vi "RamdomCOlumsFileio.vi"   [LabVIEW 2015]
types:
  T1 = enum16{"open", "replace", "create", "open or create", "replace or create", "replace or create with confirmation"}
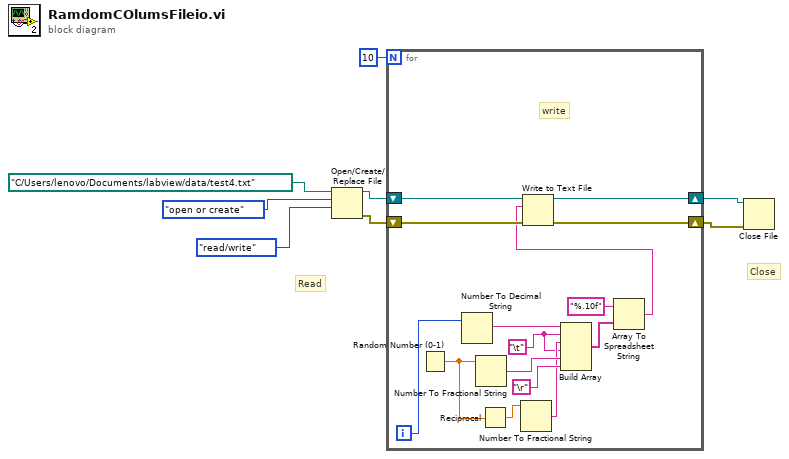
[diagram p0: block diagram]
diagram:
  # "Read"
  # "Close"
  n1 = Open/Create/Replace File(file path (use dialog)=path "C:/Users/lenovo/Documents/labview/data/test4.txt", operation (0:open)=T1."open or create", access (0:read/write)=enum16{"read/write", "read-only", "write-only"}."read/write") -> (refnum out=w4:refnum<file>, error out=w3:errorcluster)  [unwired: 3 in, 1 out]
  n2 = for {
    N: 10 -> [_]
    shift-right: [w20] -> w1
    shift-left: w4 -> [w23]
    shift-right: [w21] -> w2
    shift-left: w3 -> [w22]
    i -> [w18]
    w9 = "\t"
    # "write"
    n3 = Random Number (0-1)() -> (number: 0 to 1=w11:dbl)
    n4 = Number To Decimal String(number=w18) -> (decimal integer string=w19:string)  [unwired: 1 in]
    n5 = Number To Fractional String(number=w11) -> (F-format string=w13:string)  [unwired: 3 in]
    n6 = Reciprocal(x=w11) -> (1/x=w12:dbl)
    n7 = Number To Fractional String(number=w12) -> (F-format string=w10:string)  [unwired: 3 in]
    n8 = Build Array(w19, w9, w10, w9, w13, "\r") -> (w16:string[])
    n9 = Array To Spreadsheet String(array=w16, 3:"%.10f" ("format string")) -> (spreadsheet string=w15:string)  [unwired: 1 in]
    n10 = Write to Text File(file (use dialog)=w23, text=w15, error in=w22) -> (refnum out=w20:refnum<file>, error out=w21:errorcluster)  [unwired: 1 in, 1 out]
  }
  n11 = Close File(refnum=w1, error in=w2) -> ()  [unwired: 2 out]
